vi "SwitchToAnalogOrDigital.vi"(0 "System no.":i32=1 min=1 max=4 step=1, 1 "Controller analog board":enum16{"E-711.iA4"}(ring), 2 "Axes to command":string[](array[string]), 3 "Mode":bool=TRUE caption="Mode (Analog:T)", 5 "error in":errorcluster, 6 "AI channels":dbl[](array[numeric]), 7 "AO channels":dbl[](array[numeric]), 8 "Lower voltage limit (V)":dbl=-10.0 format="%.6f", 9 "Upper voltage limit (V)":dbl=10.0 format="%.6f") -> (14 "Conversion factor":dbl[](array[numeric]) format="%.2f", 15 "Offset":dbl[](array[numeric]) format="%#.6f", 19 "Error out":errorcluster)   [LabVIEW 2015]
doc: "This VI sets communication parameters for analog or digital control. Run XXXX_Configuration_Setup.vi (with XXXX being the product number of your PI controller) prior to running this VI. \n\n¢ Set System no. to the same value as selected in XXXX_Configuration_ Setup.vi. \n¢ Select the name of the controller analog board (E-711.iA4).\n¢ Mode can be Analog (T) or Digital (F). \n¢ Lower voltage limit (V) and Upper voltage limit (V) must match the corresponding settings in Analog_Configuration_Setup.vi, representing the voltage range of the analog input of the controller. The VI checks if the selected values fit into the analog input voltage range of the controller. \n¢ Axes to command must be a sub set of the axes connected to the controller. \n¢ AI channels are the analog input channels of the controller to use for analog control. In contrast to the firmware internal names of the analog input channels, select \"1\" here for the first analog input, \"2\" for the second and so on. The VI will automatically determine which input channel names correspond to the selected analog input channels. \n¢ Similarly, select \"1\" for the first analog output channel (AO channels), \"2\" for the second analog output channel and so on, as the VI will automatically determine which output channel names correspond to the selected analog output channels. \n\nIf the current command level is 0 (CCL?), the VI switches to command level 1 (CCL) before making any further settings and back to 0 afterwards. \nWhen Analog is selected as Mode, the VI connects the selected analog input channels to the selected axes (SPA), sets gain and offset for the analog input (SPA), sets the output type to sensor monitor output (SPA), connects the selected analog output channels to the selected axes (SPA), and sets the position report scaling value and offset for the analog output (SPA).\nWhen Digital is selected as Mode, the VI disconnects the selected analog input channels from the axes (SPA) and sets the output type to control output (SPA).\nThe VI returns the total number of input and output channels available for this controller, the number of sensor input/output channels and the resulting number of analog input/output channels available for analog control. Also, it returns the Gain, Offset and Conversion factor settings resulting from the motion range (TMX?, TMN?) of the selected axes and sets the corresponding parameters (SPA). Finally, it returns the minimum and maximum analog input voltages of the controller as the given lower and upper voltage limits must fit into this range.\n\nSee XXXX_Sample_Application_With_Analog.vi (with XXXX being the product number of your PI controller) as a sample VI showing how to use this VI in combination with the corresponding Configuration_Setup VIs. \n\nValid for: E-712, E-725\n\nE-712: Controller analog board is E-711.iA\nE-725: Controller analog board selection is E-711.iA (but board has different product code)."
panel:
  out "Max. controller\nanalog input voltage":dbl format="%#.6f"
  out "Min. controller\nanalog input voltage":dbl format="%#.6f"
  out "Gain":dbl[](array[numeric]) format="%#.6f"
  out "No. of output channels":dbl format="%#.0f"
  out "No. of sensor output channels":dbl format="%#.0f"
  out "No. of AO channels":dbl format="%#.0f"
  out "No. of AI channels":dbl format="%#.0f"
  out "No. of sensor input channels":dbl format="%#.0f"
  out "No. of input channels":dbl format="%#.0f"
  # "This VI sets communication parameters for analog or digital control. Run XXXX_Configuration_Setup.vi (with XXXX being the \nproduct number of your PI controller) prior to running this VI. Set System no. to the same value as selected in XXXX_Configu-\nration_Setup.vi. See online help for details."
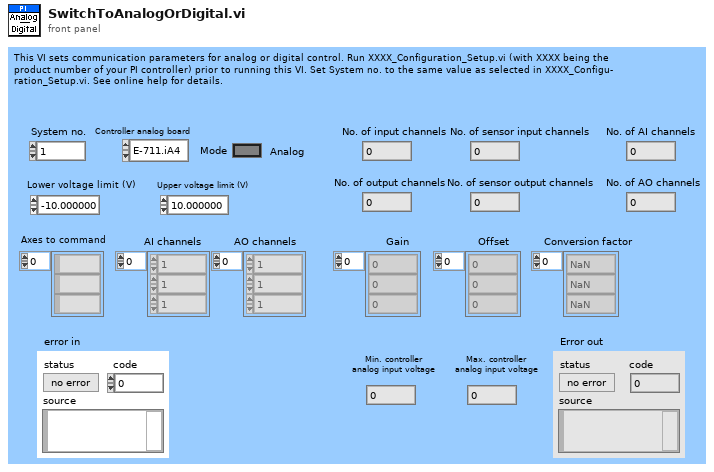
[diagram p1: front panel]
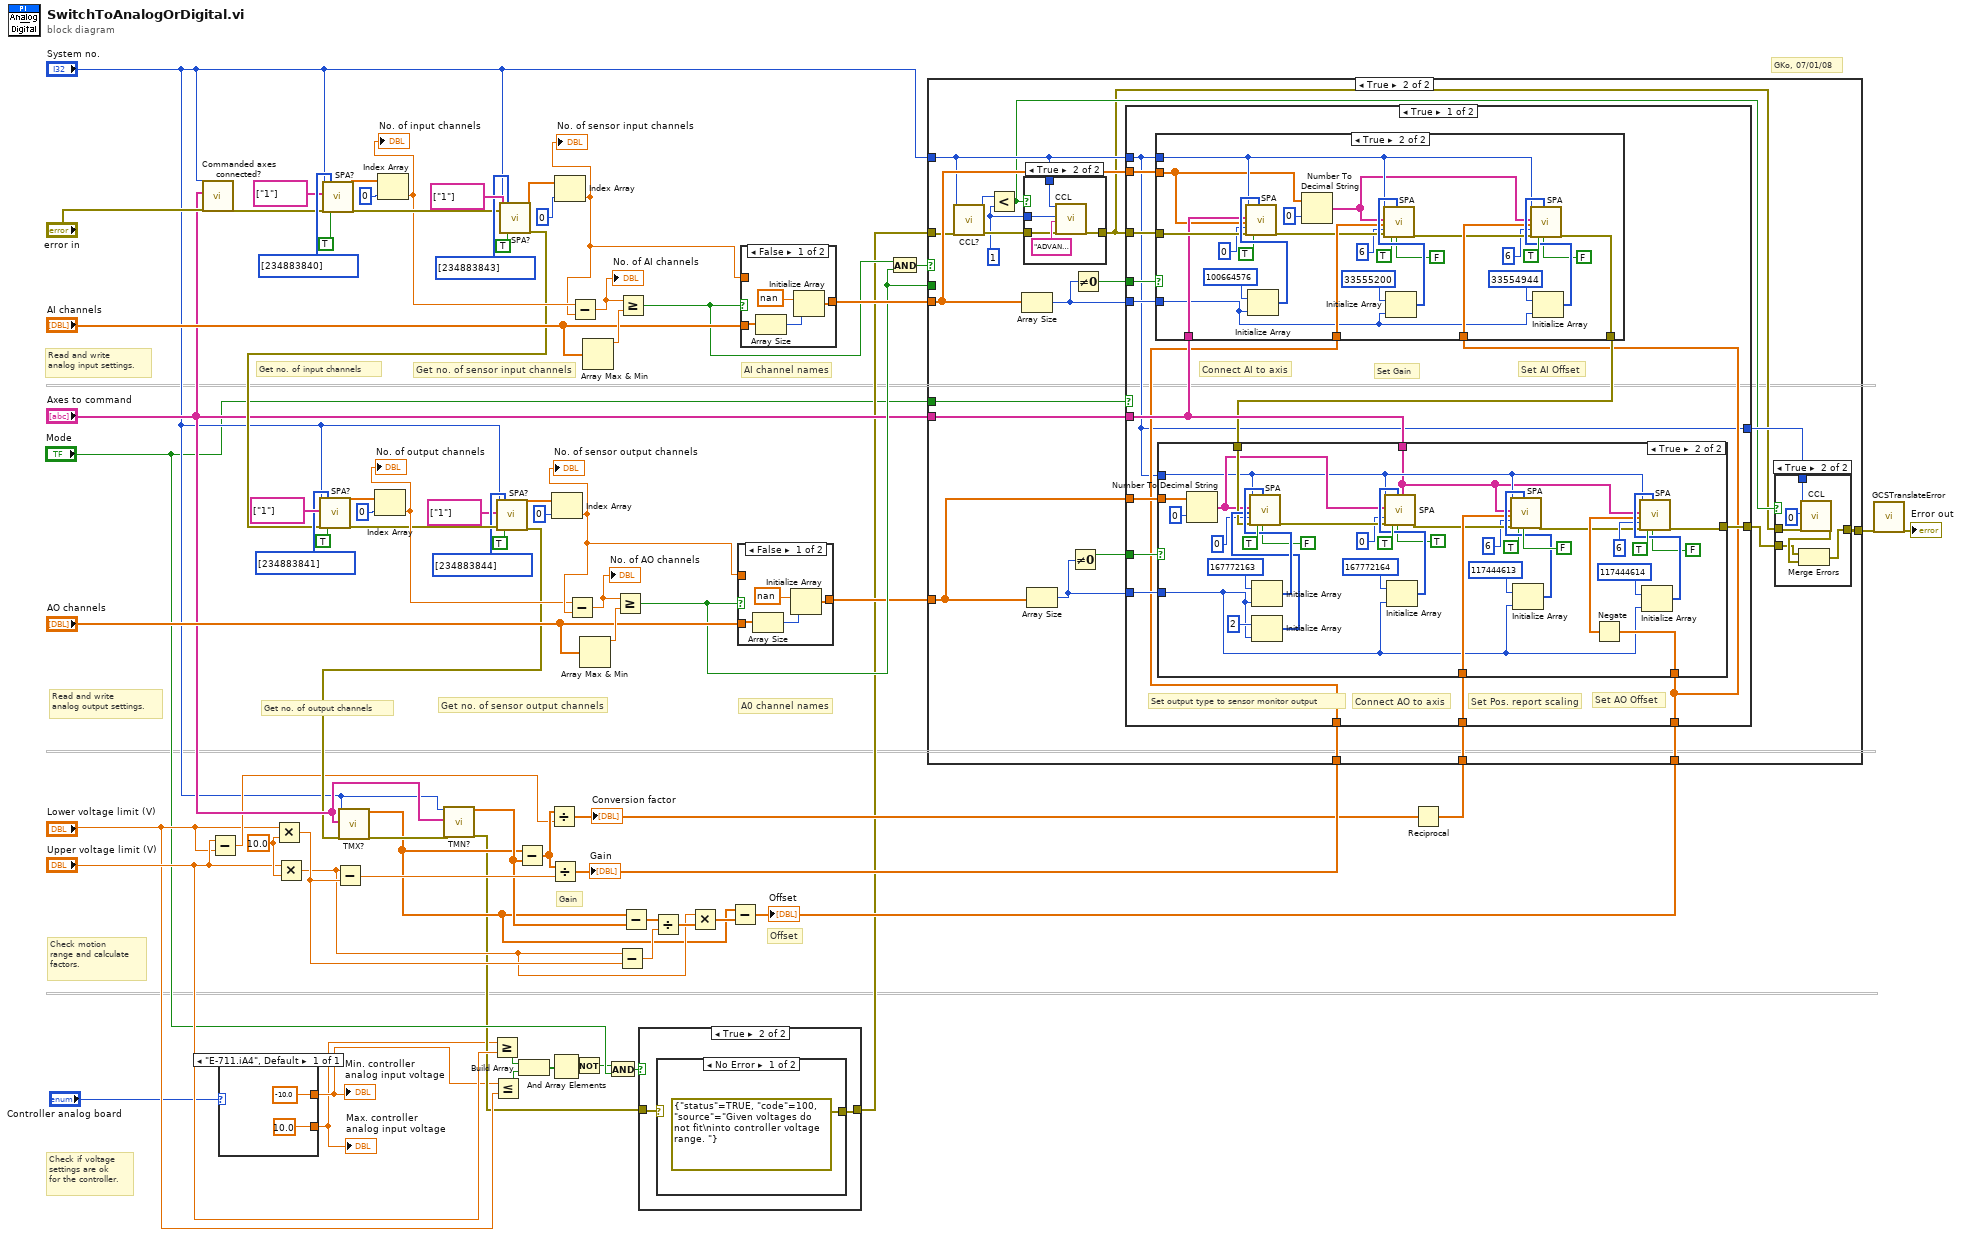
[diagram p0: block diagram]
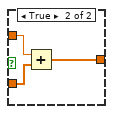
[diagram p4: hidden frame]
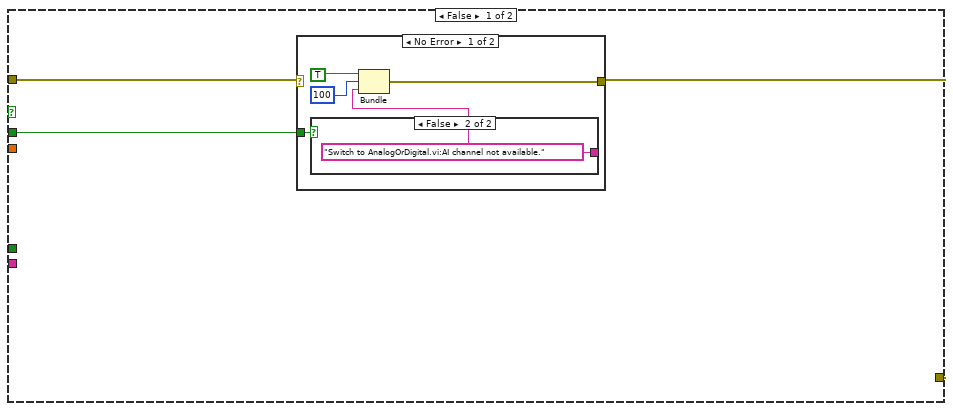
[diagram p5: hidden frame]
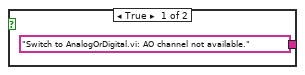
[diagram p6: hidden frame]
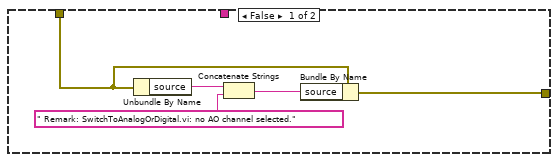
[diagram p10: hidden frame]
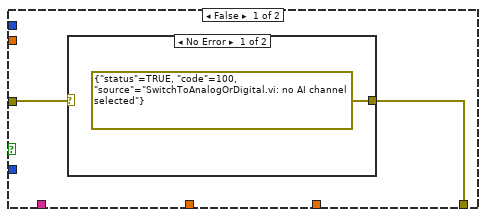
[diagram p11: hidden frame]
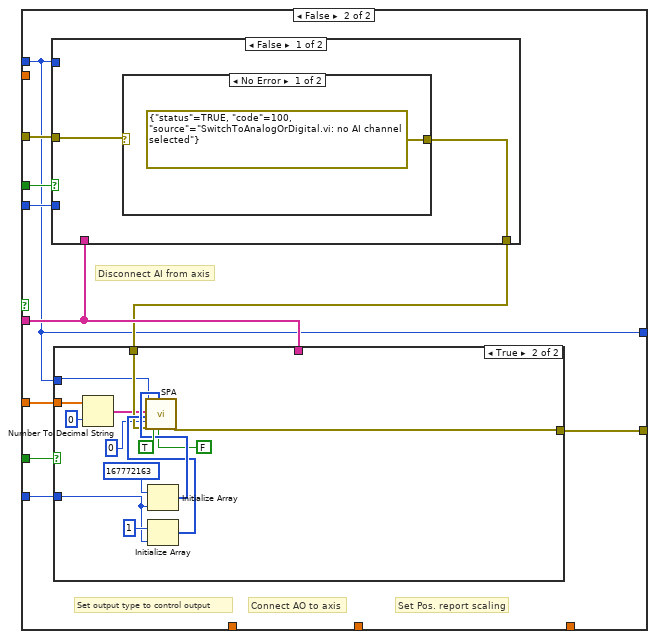
[diagram p13: hidden frame]
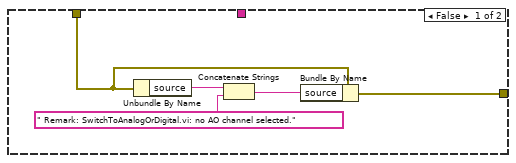
[diagram p14: hidden frame]
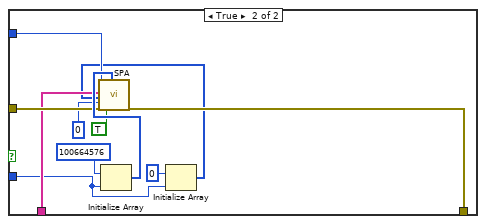
[diagram p16: hidden frame]
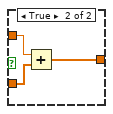
[diagram p17: hidden frame]
diagram:
  w37 = 10.0 ("y")
  # "Get no. of sensor output channels"
  # "Get no. of output channels"
  # "Get no. of sensor input channels"
  # "Get no. of input channels"
  # "Offset"
  # "Gain"
  # "A0 channel names"
  # "GKo, 07/01/08"
  # "Read and write\nanalog output settings."
  # "Check motion\nrange and calculate\nfactors."
  # "Check if voltage\nsettings are ok\nfor the controller."
  # "AI channel names"
  # "Read and write\nanalog input settings."
  n1 = call "Commanded axes connected?.vi"("System no."="System no.", "Commanded axes"="Axes to command", "error in"="error in") -> ("error out"=w60:errorcluster)  [unwired: 15 in, 1 out]
  n2 = Subtract(x="Upper voltage limit (V)", y="Lower voltage limit (V)") -> (x-y=w21:dbl)
  n3 = case shown="\"E-711.iA4\", Default" "Controller analog board" {
    tunnel: [-10.0 ("y")] -> w3
    tunnel: [10.0 ("y")] -> w2
    frame "E-711.iA4", Default {
    }
  }
  "Min. controller\nanalog input voltage" <- w3
  "Max. controller\nanalog input voltage" <- w2
  n4 = Multiply(x="Lower voltage limit (V)", y=w37) -> (x*y=w32:dbl)
  n5 = Multiply(x="Upper voltage limit (V)", y=w37) -> (x*y=w27:dbl)
  n6 = call "SPA?.vi"("System no."="System no.", "Axes to query"=string[] ["1"], "error in"=w60, "Parameter no. (hex)"=u32[] [234883840], "Parameter no. format \n(Decimal: FALSE)"=TRUE ("Parameter no. format \n(Decimal: FALSE)")) -> ("Parameter value"=w73:dbl[], "error out"=w66:errorcluster)  [unwired: 9 in, 4 out]
  n7 = Subtract(x=w27, y=w32) -> (x-y=w33:dbl)
  n8 = Index Array(array=w73, index=0) -> (element=w65:dbl)
  "No. of input channels" <- w65
  n9 = Greater Or Equal?(x=w2, y="Upper voltage limit (V)") -> (x >= y?=w14:bool)
  n10 = Less Or Equal?(x=w3, y="Lower voltage limit (V)") -> (x <= y?=w13:bool)
  n11 = call "SPA?.vi"("System no."="System no.", "Axes to query"=string[] ["1"], "error in"=w66, "Parameter no. (hex)"=u32[] [234883843], "Parameter no. format \n(Decimal: FALSE)"=TRUE ("Parameter no. format \n(Decimal: FALSE)")) -> ("Parameter value"=w70:dbl[], "error out"=w42:errorcluster)  [unwired: 9 in, 4 out]
  n12 = call "SPA?.vi"("System no."="System no.", "Axes to query"=string[] ["1"], "error in"=w42, "Parameter no. (hex)"=u32[] [234883841], "Parameter no. format \n(Decimal: FALSE)"=TRUE ("Parameter no. format \n(Decimal: FALSE)")) -> ("Parameter value"=w46:dbl[], "error out"=w53:errorcluster)  [unwired: 9 in, 4 out]
  n13 = Index Array(array=w46, index=0) -> (element=w54:dbl)
  "No. of output channels" <- w54
  n14 = call "SPA?.vi"("System no."="System no.", "Axes to query"=string[] ["1"], "error in"=w53, "Parameter no. (hex)"=u32[] [234883844], "Parameter no. format \n(Decimal: FALSE)"=TRUE ("Parameter no. format \n(Decimal: FALSE)")) -> ("Parameter value"=w49:dbl[], "error out"=w35:errorcluster)  [unwired: 9 in, 4 out]
  n15 = call "TMX?.vi"("System no."="System no.", "Axes to query"="Axes to command", "error in"=w35) -> ("Maximum travel limit"=w25:dbl[], "error out"=w34:errorcluster)  [unwired: 15 in]
  n16 = call "TMN?.vi"("System no."="System no.", "Axes to query"="Axes to command", "error in"=w34) -> ("Minimum travel limit"=w31:dbl[], "error out"=w4:errorcluster)  [unwired: 15 in]
  n17 = Subtract(x=w25, y=w31) -> (x-y=w22:dbl[])
  n18 = Build Array(w14, w13) -> (w12:bool[])
  n19 = Divide(x=w22, y=w21) -> (x/y=w20:dbl[])
  "Conversion factor" <- w20
  n20 = Divide(x=w22, y=w33) -> (x/y=w24:dbl[])
  "Gain" <- w24
  n21 = And Array Elements(Boolean array=w12) -> (logical AND=w8:bool)
  n22 = Index Array(array=w49, index=0) -> (element=w55:dbl)
  "No. of sensor output channels" <- w55
  n23 = Index Array(array=w70, index=0) -> (element=w64:dbl)
  "No. of sensor input channels" <- w64
  n24 = Subtract(x=w54, y=w55) -> (x-y=w56:dbl)
  "No. of AO channels" <- w56
  n25 = Subtract(x=w65, y=w64) -> (x-y=w63:dbl)
  "No. of AI channels" <- w63
  n26 = Not(x=w8) -> (.not. x?=w6:bool)
  n27 = Array Max & Min(array="AO channels") -> (max value=w57:dbl)  [unwired: 3 out]
  n28 = Array Max & Min(array="AI channels") -> (max value=w62:dbl)  [unwired: 3 out]
  n29 = And(x=w6, y="Mode") -> (x .and. y?=w5:bool)
  n30 = Greater Or Equal?(x=w56, y=w57) -> (x >= y?=w38:bool)
  n31 = Subtract(x=w27, y=w32) -> (x-y=w29:dbl)
  n32 = Greater Or Equal?(x=w63, y=w62) -> (x >= y?=w40:bool)
  n33 = Subtract(x=w25, y=w31) -> (x-y=w30:dbl[])
  n34 = case shown="True" w5 {
    tunnel: w4 -> [w79 w81]
    tunnel: [w79 w80] -> w11
    frame False {
    }
    frame True {
      n35 = case shown="No Error" w81 {
        selector: w81 -> [_ w83]
        tunnel: [errorcluster {"status"=TRUE, "code"=100, "source"="Given voltages do not fit\ninto controller voltage range. "} ("error IO") w83] -> w80
        frame No Error {
        }
        frame Error {
        }
      }
    }
  }
  n36 = Divide(x=w30, y=w29) -> (x/y=w28:dbl[])
  n37 = Multiply(x=w27, y=w28) -> (x*y=w26:dbl[])
  n38 = Subtract(x=w25, y=w26) -> (x-y=w23:dbl[])
  "Offset" <- w23
  n39 = case shown="False" w38 {
    tunnel: "AO channels" -> [w87 w89]
    tunnel: w55 -> [_ w90]
    tunnel: [w84 w88] -> w18
    frame False {
      n40 = Array Size(array=w87) -> (size(s)=w85:i32)
      n41 = Initialize Array(nan, w85) -> (w84:dbl[])
    }
    frame True {
      n42 = Add(x=w90, y=w89) -> (x+y=w88:dbl[])
    }
  }
  n43 = case shown="False" w40 {
    tunnel: "AI channels" -> [w94 w96]
    tunnel: w64 -> [_ w97]
    tunnel: [w91 w95] -> w58
    frame False {
      n44 = Array Size(array=w94) -> (size(s)=w92:i32)
      n45 = Initialize Array(nan, w92) -> (w91:dbl[])
    }
    frame True {
      n46 = Add(x=w97, y=w96) -> (x+y=w95:dbl[])
    }
  }
  n47 = And(x=w40, y=w38) -> (x .and. y?=w39:bool)
  n48 = Reciprocal(x=w20) -> (1/x=w19:dbl[])
  n49 = case shown="True" w39 {
    tunnel: "System no." -> [_ w114]
    tunnel: w58 -> [_ w119]
    tunnel: "Axes to command" -> [_ w128]
    tunnel: w11 -> [w100 w115]
    tunnel: w38 -> [w99 _]
    tunnel: w18 -> [_ w129]
    tunnel: w24 -> [_ w122]
    tunnel: w23 -> [_ w121]
    tunnel: [w98 w118] -> w10
    tunnel: w19 -> [_ w127]
    tunnel: "Mode" -> [_ w120]
    frame False {
      n50 = case shown="No Error" w100 {
        selector: w100 -> [_ w108]
        tunnel: w99 -> [w103 _]
        tunnel: [w101 w108] -> w98
        frame No Error {
          n51 = case shown="False" w103 {
            tunnel: ["Switch to AnalogOrDigital.vi: AO channel not available." ("source") "Switch to AnalogOrDigital.vi:AI channel not available." ("source")] -> w102
            frame True {
            }
            frame False {
            }
          }
          n52 = Bundle("status"=TRUE, "code"=100, "source"=w102) -> (w101:errorcluster)  [unwired: 1 in]
        }
        frame Error {
        }
      }
    }
    frame True {
      w112 = 1 ("Command level")
      n53 = call "CCL?.vi"("System no."=w114, "error in"=w115) -> ("Command level"=w113:i32, "error out"=w116:errorcluster)  [unwired: 16 in]
      n54 = Less?(x=w113, y=w112) -> (x < y?=w111:bool)
      n55 = Array Size(array=w119) -> (size(s)=w125:i32)
      n56 = case shown="True" w111 {
        tunnel: [w137 w142] -> w110
        tunnel: w116 -> [w137 w140]
        tunnel: w114 -> [_ w139]
        tunnel: w112 -> [_ w138]
        frame False {
        }
        frame True {
          n57 = call "CCL.vi"("System no."=w139, "Command level"=w138, "Password"="ADVANCED", "error in"=w140) -> ("error out"=w142:errorcluster)  [unwired: 14 in, 1 out]
        }
      }
      n58 = Array Size(array=w129) -> (size(s)=w124:i32)
      n59 = Not Equal To 0?(x=w124) -> (x != 0?=w123:bool)
      n60 = Not Equal To 0?(x=w125) -> (x != 0?=w126:bool)
      n61 = case shown="True" w120 {
        tunnel: w110 -> [w156 w237]
        tunnel: w129 -> [w155 w236]
        tunnel: [w154 w235] -> w109
        tunnel: w128 -> [w153 w234]
        tunnel: w127 -> [w152 _]
        tunnel: w114 -> [w143 w228]
        tunnel: w119 -> [w150 _]
        tunnel: w126 -> [w149 w232]
        tunnel: w125 -> [w148 w231]
        tunnel: w124 -> [w147 w230]
        tunnel: w123 -> [w146 w229]
        tunnel: w122 -> [w145 _]
        tunnel: w121 -> [w144 _]
        tunnel: [w143 w228] -> w117
        frame True {
          # "Set AO Offset"
          # "Set Pos. report scaling"
          # "Set AI Offset"
          # "Set Gain"
          # "Connect AO to axis"
          # "Set output type to sensor monitor output"
          # "Connect AI to axis"
          n62 = case shown="True" w149 {
            tunnel: w156 -> [w199 w225]
            tunnel: w145 -> [_ w220]
            tunnel: w144 -> [_ w214]
            tunnel: w153 -> [_ w212]
            tunnel: [w198 w210] -> w151
            tunnel: w143 -> [_ w209]
            tunnel: w148 -> [_ w208]
            tunnel: w150 -> [_ w205]
            frame False {
              n63 = case shown="No Error" w199 {
                selector: w199 -> [_ w201]
                tunnel: [errorcluster {"status"=TRUE, "code"=100, "source"="SwitchToAnalogOrDigital.vi: no AI channel selected"} ("error IO") w201] -> w198
                frame No Error {
                }
                frame Error {
                }
              }
            }
            frame True {
              n64 = Initialize Array(100664576 ("Numeric"), w208) -> (w226:i32[])
              n65 = call "SPA.vi"("System no."=w209, "Axis to set"=w212, "Parameter value"=w205, "No.of digits"=i16 0, "error in"=w225, "Parameter no. format \n(Decimal: FALSE)"=TRUE ("Parameter no. format \n(Decimal: FALSE)"), "Parameter number (hex)"=w226) -> ("error out"=w211:errorcluster)  [unwired: 11 in, 1 out]
              n66 = Number To Decimal String(number=w205, width (-)=i16 0) -> (decimal integer string=w206:string[])
              n67 = Initialize Array(33555200 ("Numeric"), w208) -> (w222:i32[])
              n68 = call "SPA.vi"("System no."=w209, "Axis to set"=w206, "Parameter value"=w220, "No.of digits"=i16 6, "error in"=w211, "Parameter no. format \n(Decimal: FALSE)"=TRUE ("Parameter no. format \n(Decimal: FALSE)"), "Parameter number (hex)"=w222, "Parameter format \n(Num.: FALSE)"=FALSE ("Parameter format \n(Num.: FALSE)")) -> ("error out"=w213:errorcluster)  [unwired: 10 in, 1 out]
              n69 = Initialize Array(33554944 ("Numeric"), w208) -> (w218:i32[])
              n70 = call "SPA.vi"("System no."=w209, "Axis to set"=w206, "Parameter value"=w214, "No.of digits"=i16 6, "error in"=w213, "Parameter no. format \n(Decimal: FALSE)"=TRUE ("Parameter no. format \n(Decimal: FALSE)"), "Parameter number (hex)"=w218, "Parameter format \n(Num.: FALSE)"=FALSE ("Parameter format \n(Num.: FALSE)")) -> ("error out"=w210:errorcluster)  [unwired: 10 in, 1 out]
            }
          }
          n71 = case shown="True" w146 {
            tunnel: w155 -> [_ w189]
            tunnel: [w157 w163] -> w154
            tunnel: w153 -> [_ w170]
            tunnel: w152 -> [_ w181]
            tunnel: w151 -> [w158 w180]
            tunnel: w143 -> [_ w173]
            tunnel: w147 -> [_ w162]
            tunnel: w144 -> [_ w172]
            frame False {
              n72 = Unbundle By Name(w158) -> ("source"=w161:string)
              n73 = Concatenate Strings(w161, " Remark: SwitchToAnalogOrDigital.vi: no AO channel selected." ("source")) -> (w159:string)
              n74 = Bundle By Name(cluster=w158, "source"=w159) -> (w157:errorcluster)
            }
            frame True {
              n75 = Number To Decimal String(number=w189, width (-)=i16 0) -> (decimal integer string=w179:string[])
              n76 = Initialize Array(167772163 ("Numeric"), w162) -> (w196:i32[])
              n77 = Initialize Array(2 ("element"), w162) -> (w193:i32[])
              n78 = call "SPA.vi"("System no."=w173, "Axis to set"=w179, "Parameter value"=w193, "No.of digits"=i16 0, "error in"=w180, "Parameter no. format \n(Decimal: FALSE)"=TRUE ("Parameter no. format \n(Decimal: FALSE)"), "Parameter number (hex)"=w196, "Parameter format \n(Num.: FALSE)"=FALSE ("Parameter format \n(Num.: FALSE)")) -> ("error out"=w188:errorcluster)  [unwired: 10 in, 1 out]
              n79 = Initialize Array(167772164 ("Numeric"), w162) -> (w191:i32[])
              n80 = call "SPA.vi"("System no."=w173, "Axis to set"=w179, "No.of digits"=i16 0, "error in"=w188, "Parameter no. format \n(Decimal: FALSE)"=TRUE ("Parameter no. format \n(Decimal: FALSE)"), "Parameter number (hex)"=w191, "Parameter format \n(Num.: FALSE)"=TRUE ("Parameter format \n(Num.: FALSE)"), "Parameter string"=w170) -> ("error out"=w169:errorcluster)  [unwired: 10 in, 1 out]
              n81 = Initialize Array(117444613 ("Numeric"), w162) -> (w183:i32[])
              n82 = call "SPA.vi"("System no."=w173, "Axis to set"=w170, "Parameter value"=w181, "No.of digits"=i16 6, "error in"=w169, "Parameter no. format \n(Decimal: FALSE)"=TRUE ("Parameter no. format \n(Decimal: FALSE)"), "Parameter number (hex)"=w183, "Parameter format \n(Num.: FALSE)"=FALSE ("Parameter format \n(Num.: FALSE)")) -> ("error out"=w164:errorcluster)  [unwired: 10 in, 1 out]
              n83 = Negate(x=w172) -> (-x=w171:dbl[])
              n84 = Initialize Array(117444614 ("Numeric"), w162) -> (w176:i32[])
              n85 = call "SPA.vi"("System no."=w173, "Axis to set"=w170, "Parameter value"=w171, "No.of digits"=i16 6, "error in"=w164, "Parameter no. format \n(Decimal: FALSE)"=TRUE ("Parameter no. format \n(Decimal: FALSE)"), "Parameter number (hex)"=w176, "Parameter format \n(Num.: FALSE)"=FALSE ("Parameter format \n(Num.: FALSE)")) -> ("error out"=w163:errorcluster)  [unwired: 10 in, 1 out]
            }
          }
        }
        frame False {
          # "Set Pos. report scaling"
          # "Connect AO to axis"
          # "Set output type to control output"
          # "Disconnect AI from axis"
          n86 = case shown="False" w232 {
            tunnel: w237 -> [w258 w269]
            tunnel: w234 -> [_ w267]
            tunnel: [w257 w265] -> w233
            tunnel: w228 -> [_ w266]
            tunnel: w231 -> [_ w264]
            frame False {
              n87 = case shown="No Error" w258 {
                selector: w258 -> [_ w260]
                tunnel: [errorcluster {"status"=TRUE, "code"=100, "source"="SwitchToAnalogOrDigital.vi: no AI channel selected"} ("error IO") w260] -> w257
                frame No Error {
                }
                frame Error {
                }
              }
            }
            frame True {
              n88 = Initialize Array(100664576 ("Numeric"), w264) -> (w270:i32[])
              n89 = Initialize Array(0 ("element"), w264) -> (w262:i32[])
              n90 = call "SPA.vi"("System no."=w266, "Axis to set"=w267, "Parameter value"=w262, "No.of digits"=i16 0, "error in"=w269, "Parameter no. format \n(Decimal: FALSE)"=TRUE ("Parameter no. format \n(Decimal: FALSE)"), "Parameter number (hex)"=w270) -> ("error out"=w265:errorcluster)  [unwired: 11 in, 1 out]
            }
          }
          n91 = case shown="True" w229 {
            tunnel: w236 -> [_ w251]
            tunnel: [w238 w244] -> w235
            tunnel: w234 -> [_ _]
            tunnel: w233 -> [w242 w249]
            tunnel: w228 -> [_ w248]
            tunnel: w230 -> [_ w247]
            frame False {
              n92 = Unbundle By Name(w242) -> ("source"=w241:string)
              n93 = Concatenate Strings(w241, " Remark: SwitchToAnalogOrDigital.vi: no AO channel selected." ("source")) -> (w239:string)
              n94 = Bundle By Name(cluster=w242, "source"=w239) -> (w238:errorcluster)
            }
            frame True {
              n95 = Number To Decimal String(number=w251, width (-)=i16 0) -> (decimal integer string=w246:string[])
              n96 = Initialize Array(167772163 ("Numeric"), w247) -> (w255:i32[])
              n97 = Initialize Array(1 ("element"), w247) -> (w252:i32[])
              n98 = call "SPA.vi"("System no."=w248, "Axis to set"=w246, "Parameter value"=w252, "No.of digits"=i16 0, "error in"=w249, "Parameter no. format \n(Decimal: FALSE)"=TRUE ("Parameter no. format \n(Decimal: FALSE)"), "Parameter number (hex)"=w255, "Parameter format \n(Num.: FALSE)"=FALSE ("Parameter format \n(Num.: FALSE)")) -> ("error out"=w244:errorcluster)  [unwired: 10 in, 1 out]
            }
          }
        }
      }
      n99 = case shown="True" w111 {
        tunnel: [w130 w131] -> w118
        tunnel: w117 -> [_ w136]
        tunnel: w110 -> [_ w134]
        tunnel: w109 -> [w130 w132]
        frame False {
        }
        frame True {
          n100 = call "CCL.vi"("System no."=w136, "Command level"=0, "error in"=w134) -> ("error out"=w133:errorcluster)  [unwired: 15 in, 1 out]
          n101 = Merge Errors(w132, w133) -> (w131:errorcluster)
        }
      }
    }
  }
  n102 = call "GCSTranslateError.vi"("error in"=w10) -> ("error out"=→"Error out":errorcluster)  [unwired: 16 in, 2 out]
